vi "ShoulderGlobal.vi"() -> ()   [LabVIEW 2023]
doc: "Arm global (getters and setter stuff)"
panel:
  out "Tune_Out_Min":dbl=0.05
  out "Tune_Out_Max":dbl=0.7
  out "Tune_Err_Thresh":dbl=105.0
  out "Tune_K_Grav":dbl=0.18
  out "ShoulderLowLimitSwitch":bool
  out "ShoulderExecOnTarget":bool
  out "ShoulderPosDemandDeg":dbl
  out "ShoulderMotorOutput":dbl
  out "ShoulderCalcSpeaker_Enabled":bool
  out "ShoulderPositionDeg":dbl
  # "#TODO Shoulder global rename globals --- maybe..."
  # "#TODO Once tuned, update these defaults with tuned values."
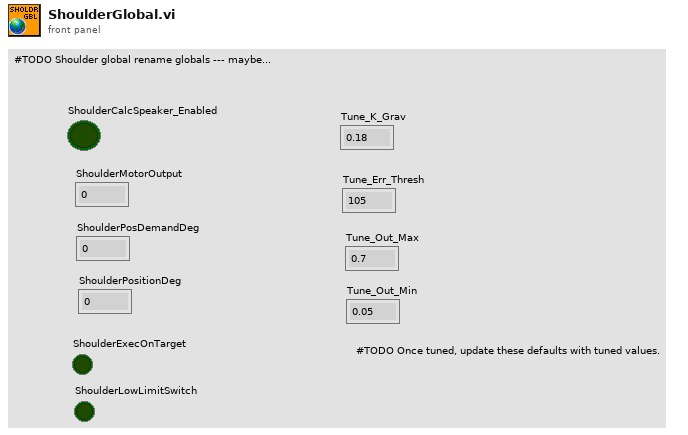
[diagram p1: front panel]
diagram:
